vi "mój.vi"() -> ()   [LabVIEW 2015]
uses:
  <vilib>/DAQmx/create/channels.llb/DAQmx Create Channel (AI-Temperature-Thermocouple).vi
  <vilib>/DAQmx/configure/timing.llb/DAQmx Timing (Sample Clock).vi
panel:
  in  "Cluster":cluster{"Thermometer":dbl, "Czêstotliwoœæ":dbl} {"Thermometer" scale=0.0..100.0}
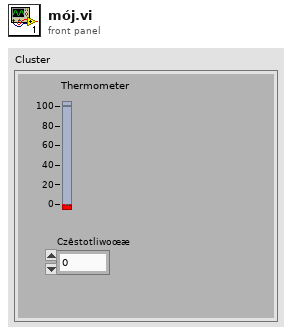
[diagram p1: front panel]
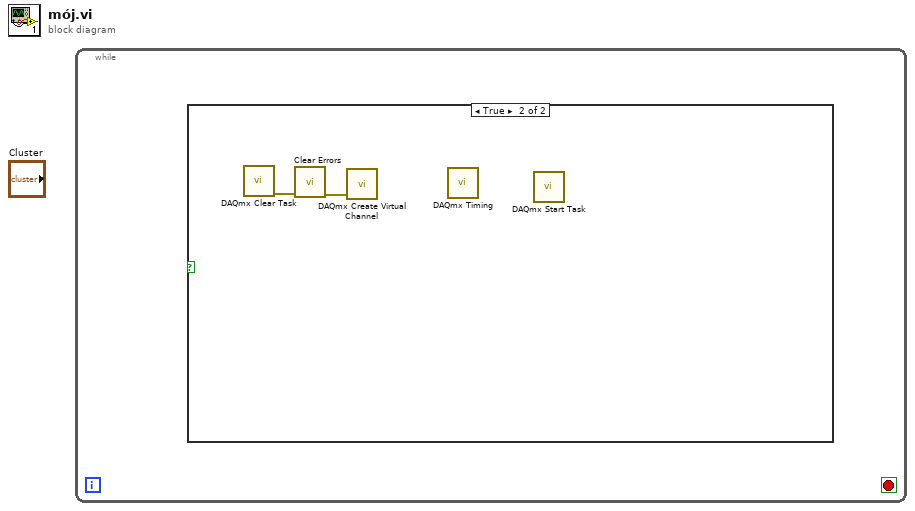
[diagram p0: block diagram]
diagram:
  n1 = while {
    stop <- _ stop-if-true
    n2 = case shown="True" {
      selector: _ -> [_ _]
      frame False {
      }
      frame True {
        n3 = call <vilib>:"DAQmx Clear Task.vi"() -> ("error out"=w2:errorcluster)  [unwired: 15 in]
        n4 = call <vilib>:"Clear Errors.vi"("error in (no error)"=w2) -> ("error out"=w1:errorcluster)  [unwired: 5 in, 1 out]
        n5 = call-poly <vilib>:"DAQmx Create Virtual Channel.vi"("error in"=w1) -> ()  [unwired: 13 in, 2 out]
        n6 = call-poly <vilib>:"DAQmx Timing.vi"() -> ()  [unwired: 14 in, 2 out]
        n7 = call <vilib>:"DAQmx Start Task.vi"() -> ()  [unwired: 14 in, 2 out]
      }
    }
  }
